vi "test debug.vi"() -> ()   [LabVIEW 2014]
panel:
  out "s":string[](array[string])
  in  "String":string
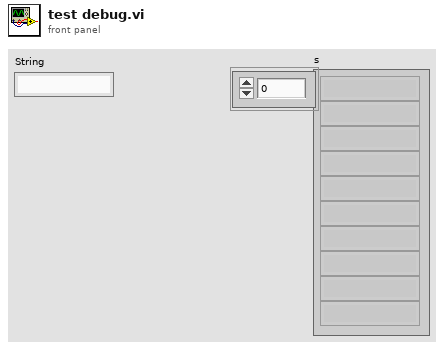
[diagram p1: front panel]
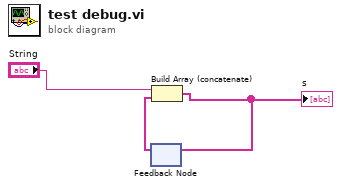
[diagram p0: block diagram]
diagram:
  n1 = feedback #1() -> (w1:string[])  [unwired: 1 in]
  n2 = Build Array (concatenate)("String", w1) -> (w2:string[])
  "s" <- w2
  n3 = feedback-in #1(w2) -> ()
